vi "Termo_1.5__.vi"() -> ()   [LabVIEW 2015]
doc: "Программа мониторинга температуры"
panel:
  out "?":bool
  out "graph_update":bool
  out "Конфиг. АЦП?":bool
  in  "Tab Control":enum32{"ИЗМЕРЕНИЯ [К]", " АЦП", "ГРАФИК"}(tab)
  in  "T2_visible":bool=TRUE
  out "T6":dbl format="%.2f"
  in  "T5_visible":bool=TRUE
  out "R5":dbl format="%.2f"
  out "T3":dbl format="%.2f"
  out "R1":dbl format="%.2f"
  out "T2":dbl format="%.2f"
  out "T5":dbl format="%.2f"
  out "R3":dbl format="%.2f"
  out "T1":dbl format="%.2f"
  out "T4":dbl format="%.2f"
  out "R2":dbl format="%.2f"
  out "R4":dbl format="%.2f"
  out "R6":dbl format="%.2f"
  in  "T1_visible":bool=TRUE
  in  "T3_visible":bool=TRUE
  in  "T4_visible":bool=TRUE
  in  "T6_visible":bool=TRUE
  in  "stop":bool
  in  "ADC_dyn_range":T1(ring)=enum."± 0.625 В"
  in  "Buf_size":u8=1 min=1 max=128
  in  "SPS":T2(ring)
  in  "IP-адрес":string="10.10.10.65"
  in  "порт":u16=4001
  in  "Очистить график":bool
  in  "load_coeff.":bool caption="Disconn"
  in  "save_coeff.":bool caption="Disconn"
  in  "Coeff_cl_ch5":T3={"k1"=19.4736079181311652, "k2"=-232.79779903171584, "k3"=1229.13228608109057005, "k4"=-3103.0388431325554801, "k5"=4219.3520172238349901, "k6"=-2697.7160155214369299, "k7"=779.55193291697651198} caption="Канал 5" {"k7" format="%#_16g"; "k6" format="%#_16g"; "k5" format="%#_16g"; "k4" format="%#_16g"; "k3" format="%#_16g"; "k2" format="%#_16g"; "k1" format="%#_16g"}
  in  "Coeff_cl_ch6":T3={"k1"=11.9061392787261866, "k2"=-139.902402561856434, "k3"=774.882810204289854, "k4"=-1837.4832512177527, "k5"=2139.5822282396256899, "k6"=-730.555961686186492, "k7"=169.810834781266749} caption="Канал 6" {"k7" format="%#_16g"; "k6" format="%#_16g"; "k5" format="%#_16g"; "k4" format="%#_16g"; "k3" format="%#_16g"; "k2" format="%#_16g"; "k1" format="%#_16g"}
  in  "GraphLookB":bool
  in  "xScale -":bool
  in  "xScale +":bool
  out "мин.":string="1"
  in  "Старт измер.":bool
  in  "Стоп измер.":bool
  in  "Добавить время":dbl(ring)=300.0 items=["10 сек."=10.0, "1 мин."=60.0, "5 мин."=300.0, "20 мин."=1200.0]
  in  "Т min":dbl=4.0 min=-10.0 max=350.0 step=0.1
  in  "Т max":dbl=300.0 min=2.0 max=500.0 step=0.1
  out "часы":string="0"
  in  "Autoscale":bool=TRUE
  out "сек.":string="0"
  out "Сутки":string
  out "счетчик":u32=4001
  in  "Запись в файл":bool
  out "Path":string
  out "refnum out":refnum<file>
  in  "header?":bool caption="Disconn"
  out "con ID":refnum<k5>
  out "Graphs T":dynamicdata(graph) caption="ТЕМПЕРАТУРА, К"
  out "Расположение файла":path
  # "Т1"
  # "T2"
  # "Т3"
  # "Т4"
  # "Сопротивление, Ом"
  # "R1"
  # "R2"
  # "R3"
  # "R4"
  # "Скорость измерений"
  # "SPS = Samples Per Second"
  # "Размер буфера усреднения"
  # "Подключение"
  # "Шкала Т"
  # "Время графика"
  # ":"
  # ":"
  # "Измерения"
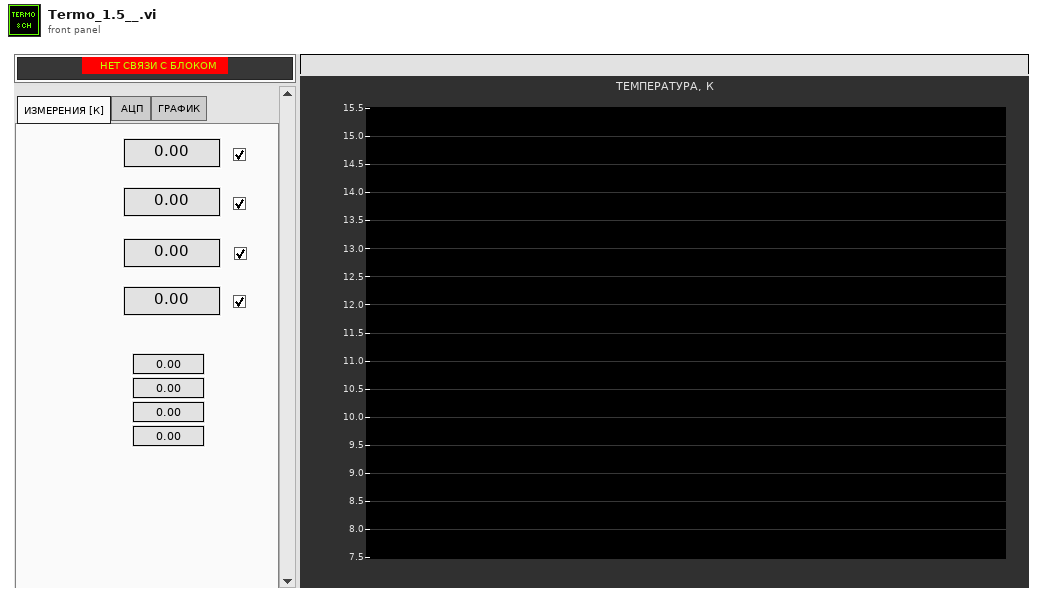
[diagram p1: front panel]
types:
  T1 = enum16{"± 5 В", "± 2.5 В", "± 1.25 В", "± 0.625 В", "± 312.5 мВ", "± 156.25 мВ", "± 78.125 мВ"}
  T2 = enum16{"2,5 SPS", "5 SPS", "10 SPS", "25 SPS", "50 SPS", "100 SPS", "500 SPS"}
  T3 = cluster{"k1":ext, "k2":ext, "k3":ext, "k4":ext, "k5":ext, "k6":ext, "k7":ext}
  T4 = enum32{"Page Enabled", "Page Disabled", "Page Disabled & Grayed"}
  T5 = enum16{"Standard", "Buffered", "CRLF", "Immediate"}
  T6 = cluster{"T1":dbl, " T2":dbl, " T3":dbl, "T4":dbl, "T5":dbl, "T6":dbl}
  T7 = typedef "LVDateTimeRec.ctl" = cluster{"fractional second":dbl, "second":i32, "minute":i32, "hour":i32, "day of month":i32, "month":i32, "year":i32, "day of week":i32, "day of year":i32, "DST":i32}
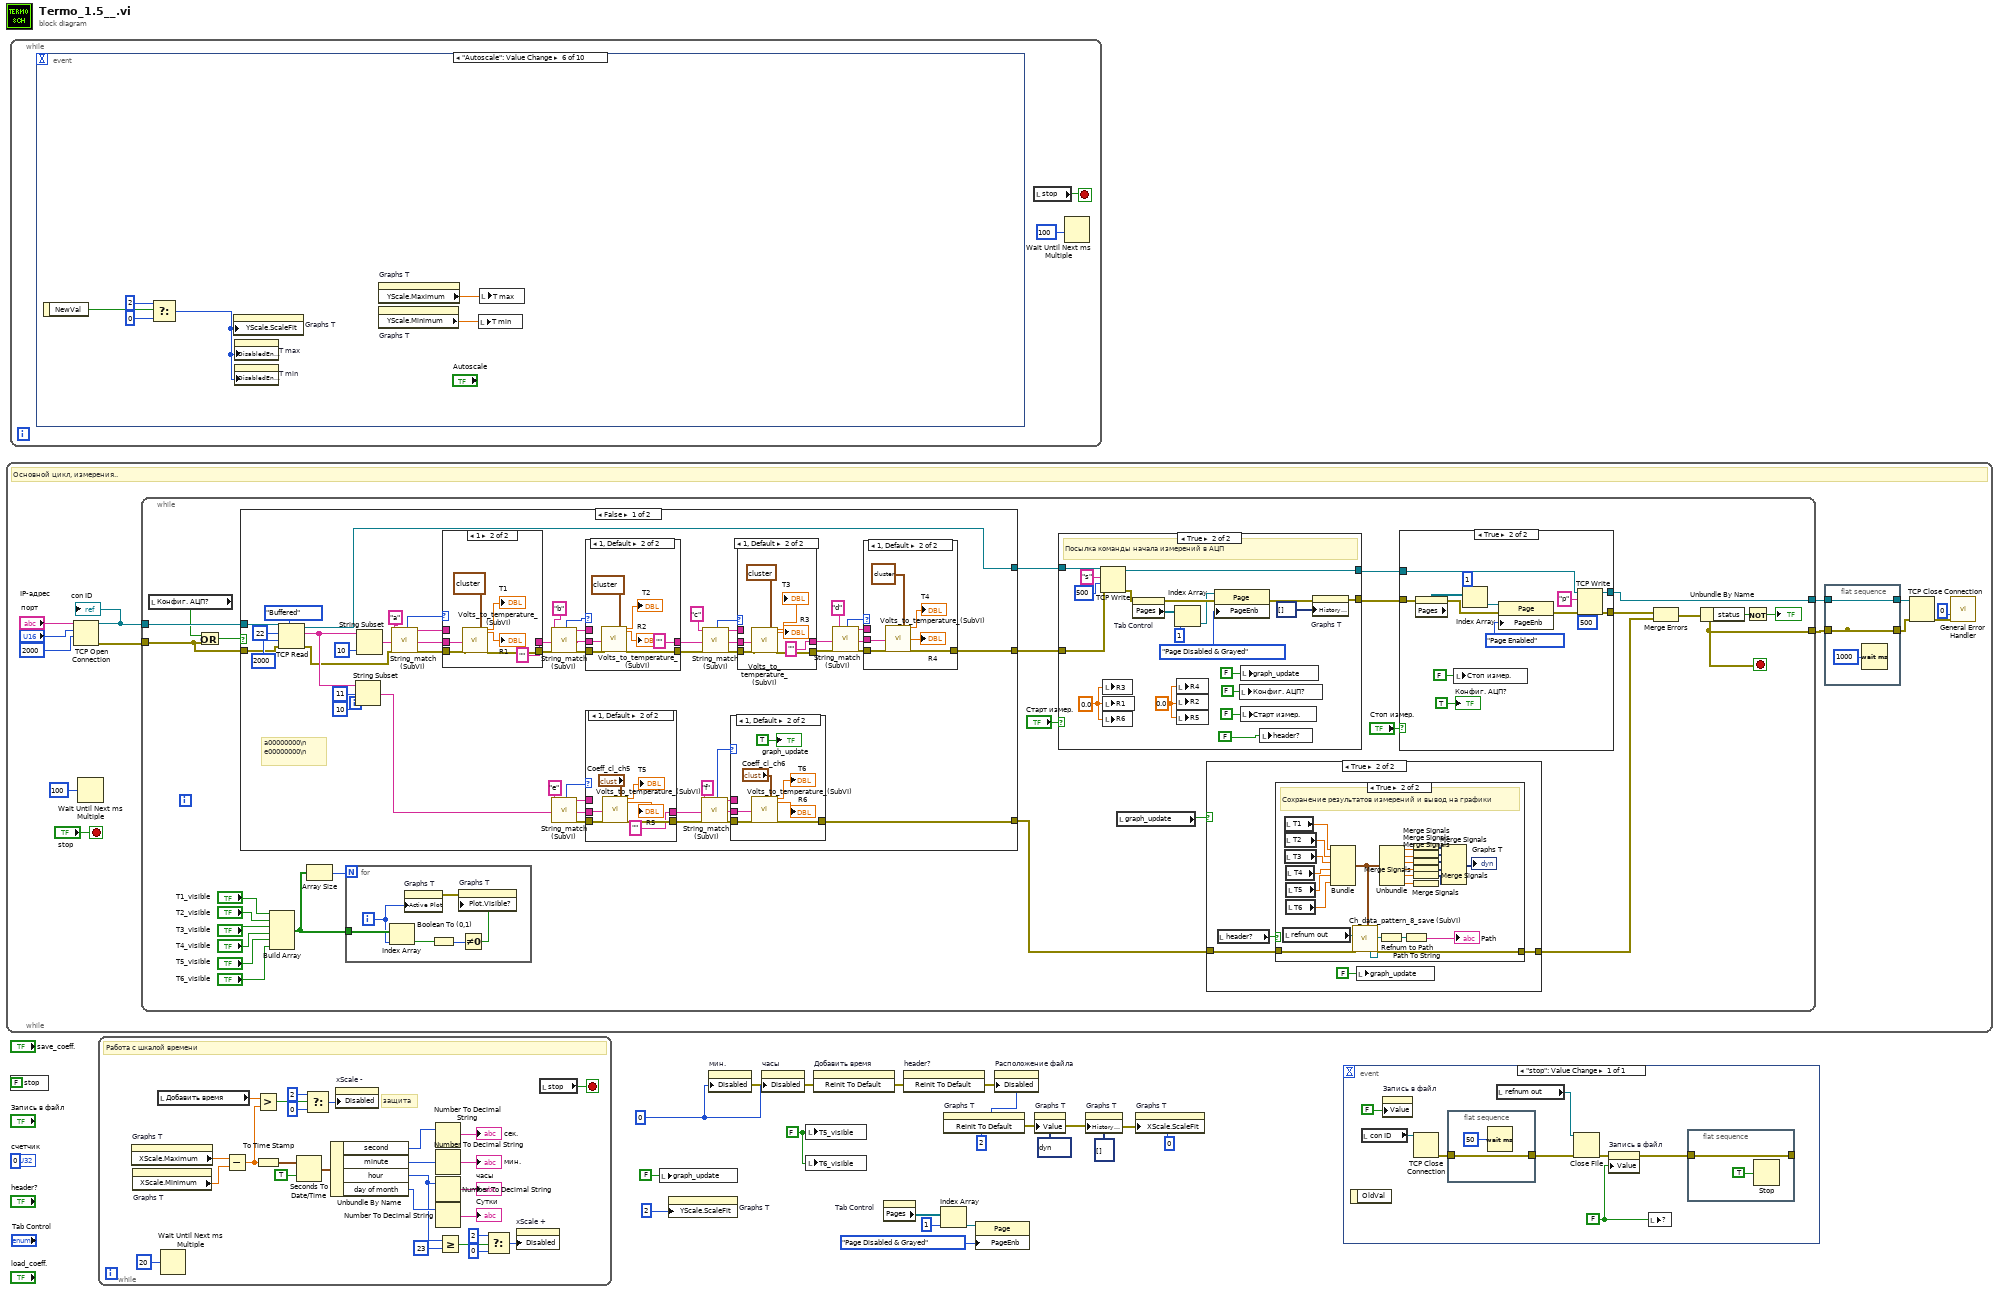
[diagram p0: block diagram]
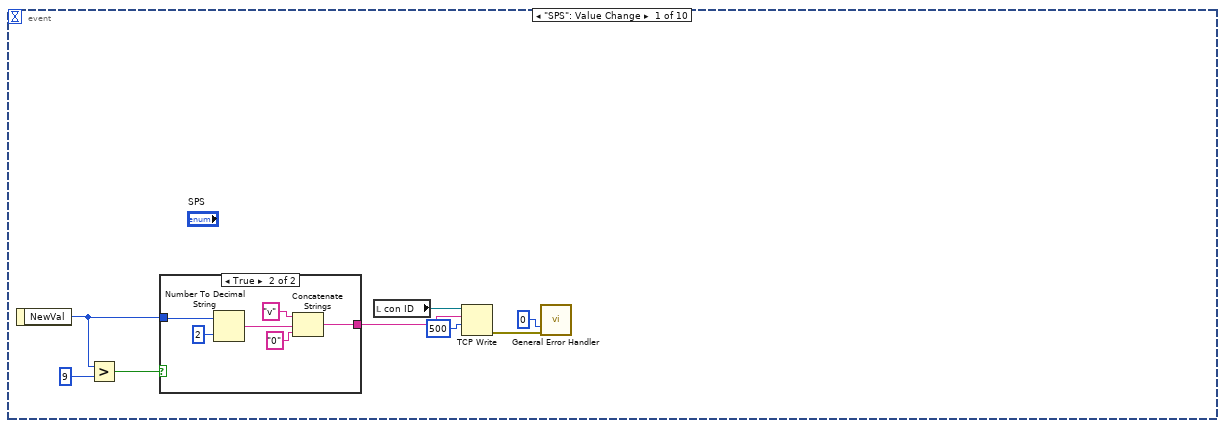
[diagram p2: hidden frame]
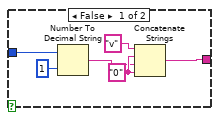
[diagram p3: hidden frame]
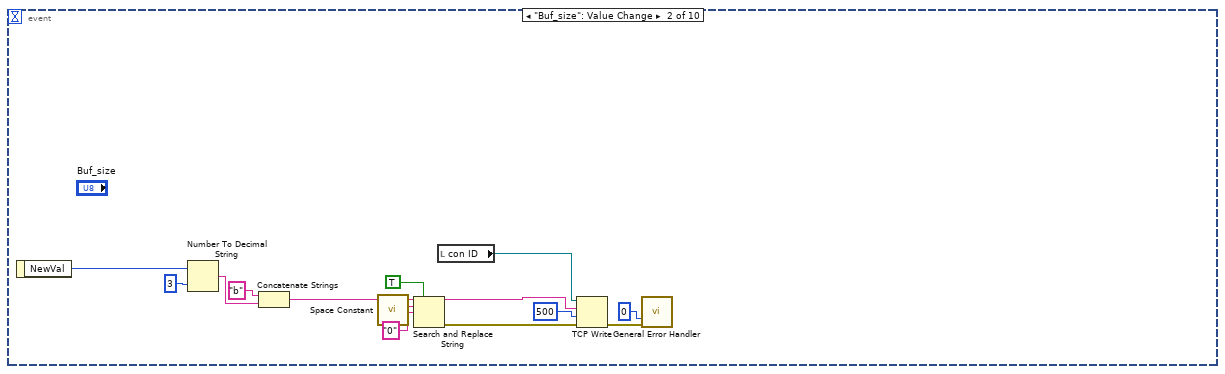
[diagram p4: hidden frame]
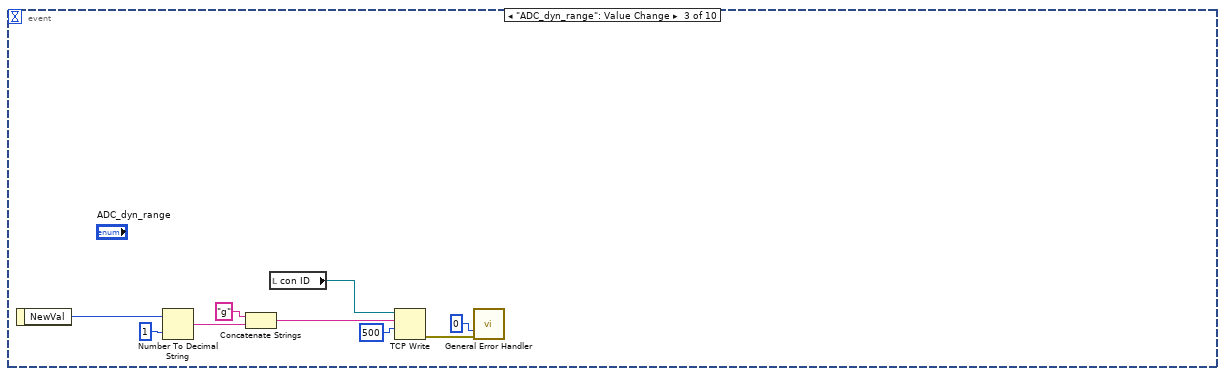
[diagram p5: hidden frame]
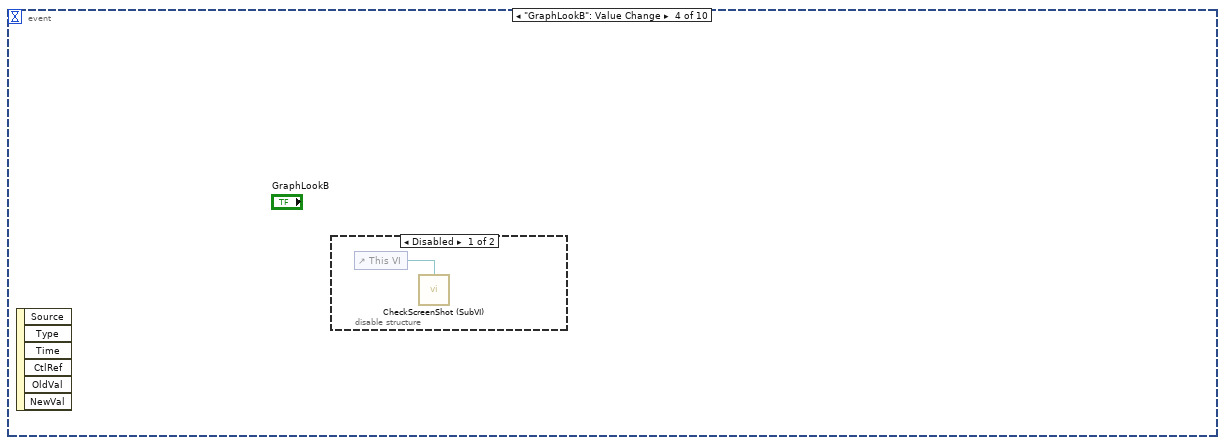
[diagram p6: hidden frame]
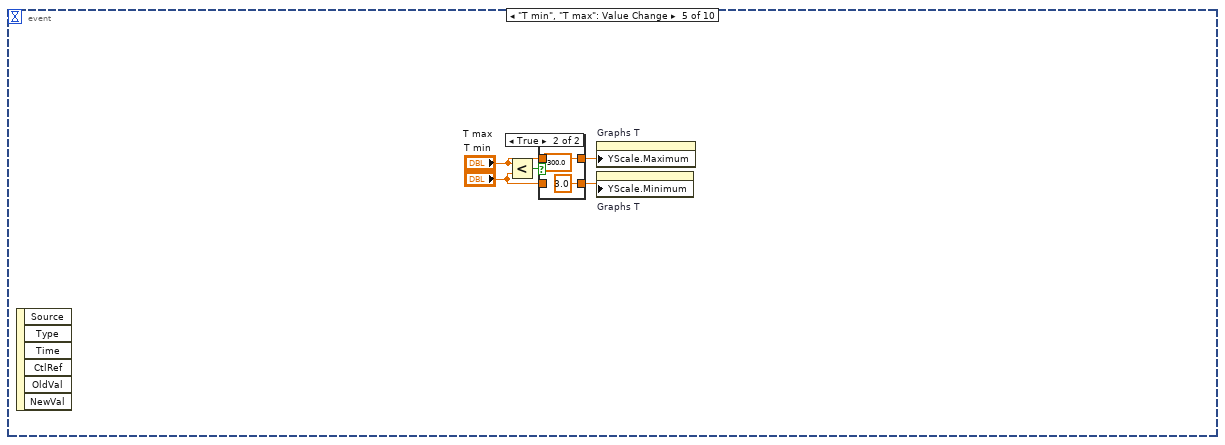
[diagram p8: hidden frame]
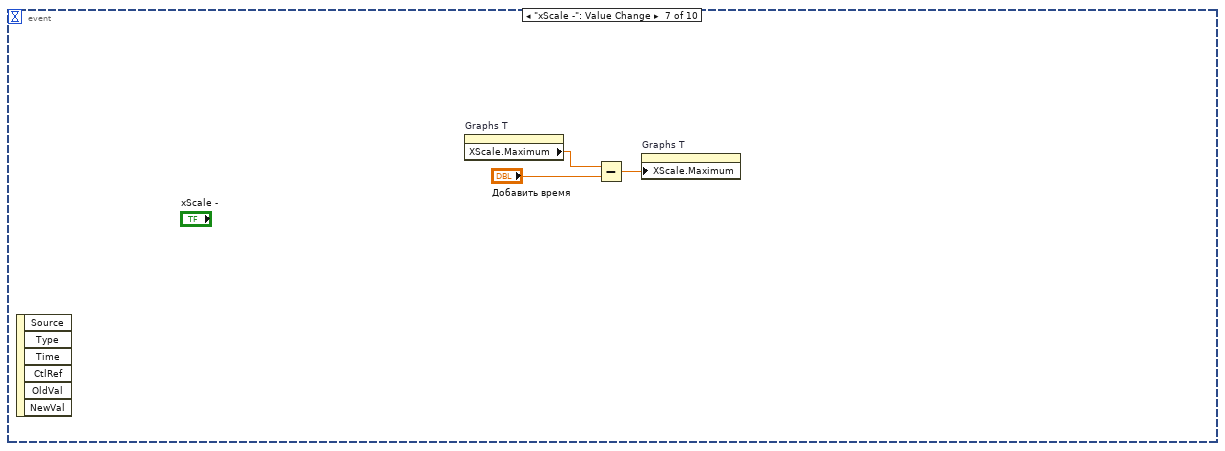
[diagram p10: hidden frame]
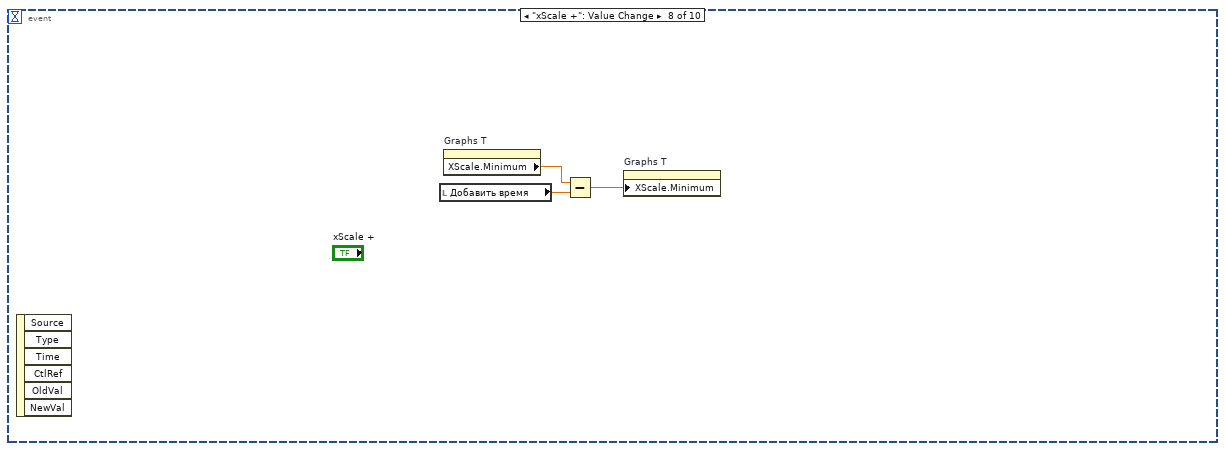
[diagram p11: hidden frame]
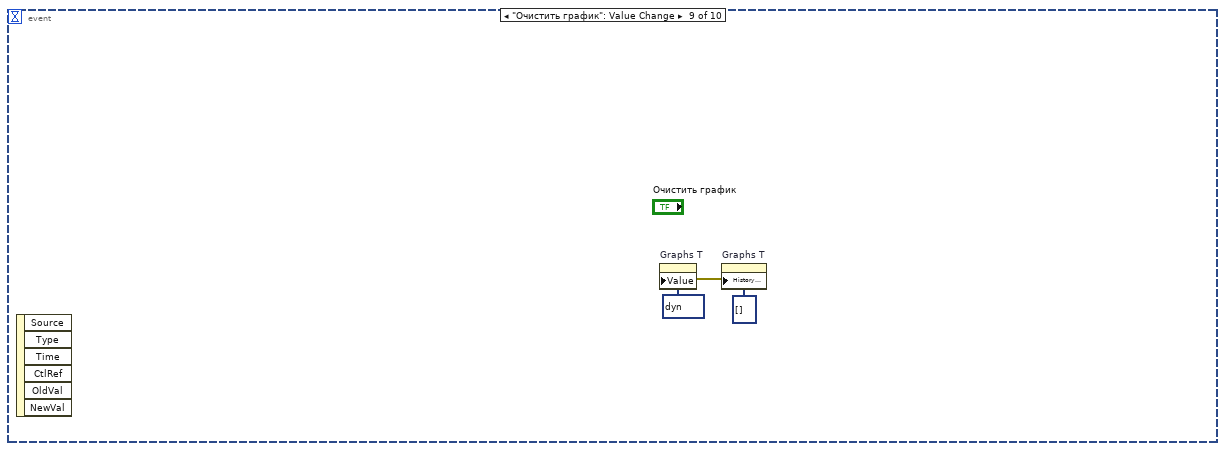
[diagram p12: hidden frame]
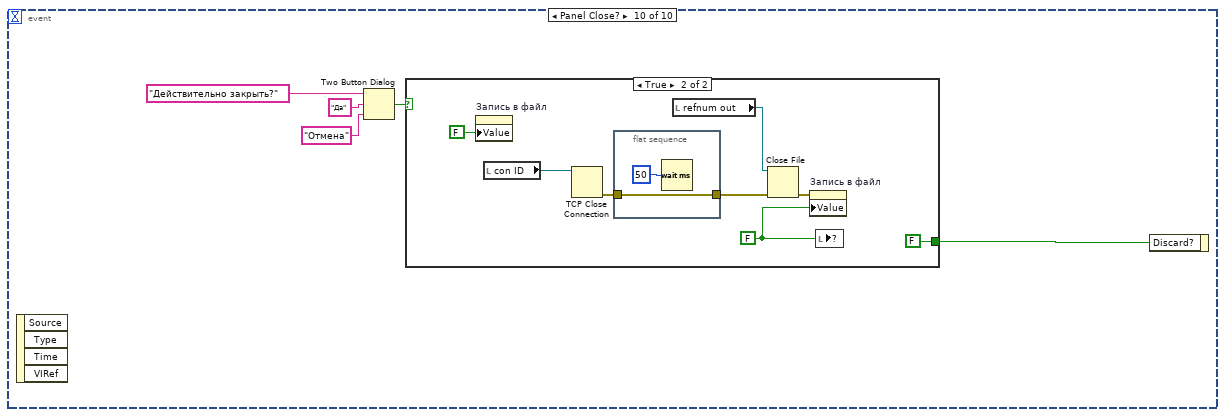
[diagram p13: hidden frame]
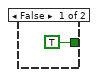
[diagram p14: hidden frame]
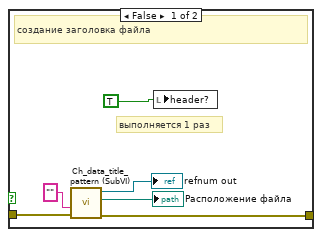
[diagram p16: hidden frame]
diagram:
  w1 = FALSE ("T5_visible")
  w20 = u8 0 ("Disabled")
  n1 = while {
    stop <- "stop" stop-if-true
    # "Основной цикл, измерения.."
    n2 = TCP Open Connection(address="IP-адрес", remote port or service name="порт", timeout ms (60000)=2000) -> (connection ID=w33:refnum<k5>, error out=w27:errorcluster)  [unwired: 1 in, 1 out]
    "con ID" <- w33
    n3 = Wait Until Next ms Multiple(millisecond multiple=u32 100) -> ()  [unwired: 1 out]
    n4 = while {
      tunnel: w33 -> [w63]
      tunnel: w27 -> [w46]
      tunnel: [w39] -> w25
      tunnel: [w38] -> w23
      stop <- w38 stop-if-true
      n5 = local read "Конфиг. АЦП?"() -> (w47:bool)
      n6 = Or(x=w47, y=w46) -> (x .or. y?=w61:bool)
      n7 = case shown="False" w61 {
        tunnel: [w146 w249] -> w48
        tunnel: w63 -> [w149 w249]
        tunnel: [w145 w248] -> w44
        tunnel: w46 -> [w147 w248]
        tunnel: [w144 _] -> w42
        frame False {
          # "a00000000\\n\ne00000000\\n"
          n8 = TCP Read(connection ID=w149, bytes to read=22, error in (no error)=w147, 7:T5."Buffered" ("mode (standard)"), 9:2000 ("timeout ms (25000)")) -> (connection ID out=w146:refnum<k5>, data out=w153:string, error out=w148:errorcluster)
          n9 = String Subset(string=w153, offset (0)=11, length (rest)=10 ("length (rest)")) -> (substring=w150:string)
          n10 = String Subset(string=w153, length (rest)=10 ("length (rest)")) -> (substring=w155:string)  [unwired: 1 in]
          n11 = call "String_match (SubVI).vi"("channel id"="a" ("regular expression"), "input string"=w155, "error in"=w148) -> ("match ?"=w161:i32, "output string"=w189:string, "match substring"=w190:string, "error out"=w191:errorcluster)  [unwired: 13 in]
          n12 = case shown="1" w161 {
            tunnel: [w240 w246] -> w180
            tunnel: w191 -> [w240 w247]
            tunnel: w190 -> [_ w245]
            tunnel: [w239 "" ("output string")] -> w193
            tunnel: w189 -> [w239 _]
            frame -1, Default {
            }
            frame 1 {
              n13 = call "Volts_to_temperature_(SubVI).vi"("ch_data_string"=w245, "error in"=w247, "koeff. cluster"=T3 {"k1"=130.445700915059999994, "k2"=-1315.82420889100000005, "k3"=5406.7587104216, "k4"=-11308.5781316600000004, "k5"=12719.274968733, "k6"=-7206.838528573, "k7"=1762.5796357467}) -> ("T solvation"=→"T1":dbl, "meas_voltage"=→"R1":dbl, "error out"=w246:errorcluster)  [unwired: 20 in, 2 out]
            }
          }
          n14 = call "String_match (SubVI).vi"("channel id"="b" ("regular expression"), "input string"=w193, "error in"=w180) -> ("match ?"=w160:i32, "output string"=w185:string, "match substring"=w186:string, "error out"=w187:errorcluster)  [unwired: 13 in]
          n15 = call "String_match (SubVI).vi"("channel id"="e" ("regular expression"), "input string"=w150) -> ("match ?"=w157:i32, "output string"=w178:string, "match substring"=w177:string, "error out"=w176:errorcluster)  [unwired: 14 in]
          n16 = case shown="1, Default" w160 {
            tunnel: [w231 w238] -> w169
            tunnel: w187 -> [w231 w237]
            tunnel: w186 -> [_ w236]
            tunnel: w185 -> [w230 _]
            tunnel: [w230 "" ("output string")] -> w168
            frame -1 {
            }
            frame 1, Default {
              n17 = call "Volts_to_temperature_(SubVI).vi"("ch_data_string"=w236, "error in"=w237, "koeff. cluster"=T3 {"k1"=158.97086338326, "k2"=-1680.987051628, "k3"=7248.2214480414, "k4"=-16012.25160649, "k5"=19138.901366204, "k6"=-11620.7677143299999996, "k7"=3012.5980224423}) -> ("T solvation"=→"T2":dbl, "meas_voltage"=→"R2":dbl, "error out"=w238:errorcluster)  [unwired: 20 in, 2 out]
            }
          }
          n18 = case shown="1, Default" w157 {
            tunnel: [w215 w222] -> w179
            tunnel: w176 -> [w215 w221]
            tunnel: w177 -> [_ w220]
            tunnel: [w214 "" ("output string")] -> w174
            tunnel: w178 -> [w214 _]
            frame -1 {
            }
            frame 1, Default {
              n19 = call "Volts_to_temperature_(SubVI).vi"("ch_data_string"=w220, "error in"=w221, "koeff. cluster"="Coeff_cl_ch5") -> ("T solvation"=→"T5":dbl, "meas_voltage"=→"R5":dbl, "error out"=w222:errorcluster)  [unwired: 20 in, 2 out]
            }
          }
          n20 = call "String_match (SubVI).vi"("channel id"="f" ("regular expression"), "input string"=w174, "error in"=w179) -> ("match ?"=w156:i32, "output string"=w173:string, "match substring"=w172:string, "error out"=w171:errorcluster)  [unwired: 13 in]
          n21 = call "String_match (SubVI).vi"("channel id"="c" ("regular expression"), "input string"=w168, "error in"=w169) -> ("match ?"=w159:i32, "output string"=w164:string, "match substring"=w165:string, "error out"=w166:errorcluster)  [unwired: 13 in]
          n22 = case shown="1, Default" w156 {
            tunnel: [w206 w213] -> w144
            tunnel: w171 -> [w206 w212]
            tunnel: w172 -> [_ w211]
            tunnel: w173 -> [_ _]
            frame -1 {
            }
            frame 1, Default {
              n23 = call "Volts_to_temperature_(SubVI).vi"("ch_data_string"=w211, "error in"=w212, "koeff. cluster"="Coeff_cl_ch6") -> ("T solvation"=→"T6":dbl, "meas_voltage"=→"R6":dbl, "error out"=w213:errorcluster)  [unwired: 20 in, 2 out]
              "graph_update" <- TRUE ("graph_update")
            }
          }
          n24 = case shown="1, Default" w159 {
            tunnel: w166 -> [w198 w205]
            tunnel: [w198 w204] -> w163
            tunnel: w165 -> [_ w202]
            tunnel: w164 -> [w197 _]
            tunnel: [w197 "" ("output string")] -> w162
            frame -1 {
            }
            frame 1, Default {
              n25 = call "Volts_to_temperature_(SubVI).vi"("ch_data_string"=w202, "error in"=w205, "koeff. cluster"=T3 {"k1"=18.933416559593, "k2"=-231.6963763814, "k3"=1256.05189673780000004, "k4"=-3242.759354941, "k5"=4499.4989483505, "k6"=-2910.138930261, "k7"=853.73352399654}) -> ("T solvation"=→"T3":dbl, "meas_voltage"=→"R3":dbl, "error out"=w204:errorcluster)  [unwired: 20 in, 2 out]
            }
          }
          n26 = call "String_match (SubVI).vi"("channel id"="d" ("regular expression"), "input string"=w162, "error in"=w163) -> ("match ?"=w158:i32, "output string"=w181:string, "match substring"=w182:string, "error out"=w183:errorcluster)  [unwired: 13 in]
          n27 = case shown="1, Default" w158 {
            tunnel: w183 -> [w223 w229]
            tunnel: [w223 w228] -> w145
            tunnel: w182 -> [_ w226]
            tunnel: w181 -> [_ _]
            frame -1 {
            }
            frame 1, Default {
              n28 = call "Volts_to_temperature_(SubVI).vi"("ch_data_string"=w226, "error in"=w229, "koeff. cluster"=T3 {"k1"=-1.22849768937512731, "k2"=42.2580823609605432, "k3"=-271.179135338868946, "k4"=1161.17997252382338, "k5"=-2451.5718683190643801, "k6"=2722.134789723902, "k7"=-982.529668014}) -> ("T solvation"=→"T4":dbl, "meas_voltage"=→"R4":dbl, "error out"=w228:errorcluster)  [unwired: 20 in, 2 out]
            }
          }
        }
        frame True {
        }
      }
      n29 = Build Array("T1_visible", "T2_visible", "T3_visible", "T4_visible", "T5_visible", "T6_visible") -> (w53:bool[])
      n30 = Array Size(array=w53) -> (size(s)=w54:i32)
      n31 = for {
        N: w54 -> [_]
        tunnel: w53 -> [w142]
        i -> [w140]
        n32 = Index Array(array=w142, index=w140) -> (element=w139:bool)
        n33 = property on="Graphs T" class="WFChart (strict)"("Active Plot"=w140) -> (error out=w141:errorcluster)  [unwired: 2 in, 1 out]
        n34 = Boolean To (0,1)(Boolean=w139) -> (0, 1=w143:i16)
        n35 = Not Equal To 0?(x=w143) -> (x != 0?=w138:bool)
        n36 = property on="Graphs T" class="WFChart (strict)"(error in=w141, "Plot.Visible?"=w138) -> ()  [unwired: 1 in, 2 out]
      }
      n37 = case shown="True" "Старт измер." {
        tunnel: [w116 w127] -> w50
        tunnel: [w117 w126] -> w52
        tunnel: w48 -> [w117 w121]
        tunnel: w44 -> [w116 w120]
        frame False {
        }
        frame True {
          w123 = 0.0 ("3")
          w118 = 0.0 ("3")
          # "Посылка команды начала измерений в АЦП"
          n38 = TCP Write(connection ID=w121, data in="s", error in (no error)=w120, 9:500 ("timeout ms (25000)")) -> (connection ID out=w126:refnum<k5>, error out=w135:errorcluster)  [unwired: 1 out]
          n39 = local write "R3"(w118) -> ()
          n40 = local write "R1"(w118) -> ()
          n41 = local write "R6"(w118) -> ()
          n42 = property on="Tab Control" class="TabCtl (strict)"(error in=w135) -> (error out=w136:errorcluster, "Pages"=w131:refnum<vi>[])  [unwired: 1 in, 1 out]
          n43 = Index Array(array=w131, index=1) -> (element=w132:refnum<vi>)
          n44 = local write "R4"(w123) -> ()
          n45 = local write "R2"(w123) -> ()
          n46 = local write "R5"(w123) -> ()
          n47 = property class="Page"(reference=w132, error in=w136, "PageEnb"=T4."Page Disabled & Grayed" ("Page Enabled State")) -> (error out=w122:errorcluster)  [unwired: 1 out]
          n48 = local write "Конфиг. АЦП?"(FALSE ("Старт измер.")) -> ()
          n49 = local write "graph_update"(FALSE ("graph_update")) -> ()
          n50 = local write "Старт измер."(FALSE ("Старт измер.")) -> ()
          n51 = local write "header?"(FALSE ("flag1")) -> ()
          n52 = property on="Graphs T" class="WFChart (strict)"(error in=w122, "History Data"=dynamicdata[] []) -> (error out=w127:errorcluster)  [unwired: 1 in, 1 out]
        }
      }
      n53 = local read "graph_update"() -> (w43:bool)
      n54 = case shown="True" w43 {
        tunnel: w42 -> [w64 w66]
        tunnel: [w64 w65] -> w40
        frame False {
        }
        frame True {
          n55 = local read "header?"() -> (w68:bool)
          n56 = case shown="True" w68 {
            tunnel: w66 -> [w69 w83]
            tunnel: [w71 w82] -> w65
            frame False {
              # "выполняется 1 раз"
              # "создание заголовка файла"
              n57 = call "Ch_data_title_pattern (SubVI).vi"("error in"=w69, "Единица измерений"="") -> ("error out"=w71:errorcluster, "Path"=→"Расположение файла":path, "Byte Stream File out"=→"refnum out":refnum<file>)  [unwired: 7 in]
              n58 = local write "header?"(TRUE ("flag1")) -> ()
            }
            frame True {
              # "Сохранение результатов измерений и вывод на графики"
              n59 = local read "refnum out"() -> (w81:refnum<file>)
              n60 = local read "T1"() -> (w80:dbl)
              n61 = local read "T2"() -> (w79:dbl)
              n62 = local read "T3"() -> (w78:dbl)
              n63 = local read "T4"() -> (w77:dbl)
              n64 = local read "T5"() -> (w76:dbl)
              n65 = local read "T6"() -> (w75:dbl)
              n66 = Bundle("T1"=w80, "T2"=w79, "T3"=w78, "T4"=w77, "T5"=w76, "T6"=w75) -> (w99:T6)  [unwired: 1 in]
              n67 = call "Ch_data_pattern_8_save (SubVI).vi"("error in"=w83, "T Cluster"=w99, "file"=w81) -> ("error out"=w82:errorcluster)  [unwired: 24 in]
              n68 = Refnum to Path(1:w81) -> (0:w98:path)
              n69 = Unbundle(w99) -> ("T1"=w91:dbl, "T2"=w90:dbl, "T3"=w89:dbl, "T4"=w88:dbl, "T5"=w86:dbl, "T6"=w84:dbl)
              n70 = Path To String(path=w98) -> (string=→"Path":string)
              n71 = Merge Signals(w91) -> (w94:dynamicdata)
              n72 = Merge Signals(w90) -> (w95:dynamicdata)
              n73 = Merge Signals(w89) -> (w96:dynamicdata)
              n74 = Merge Signals(w88) -> (w93:dynamicdata)
              n75 = Merge Signals(w86) -> (w87:dynamicdata)
              n76 = Merge Signals(w84) -> (w85:dynamicdata)
              n77 = Merge Signals(w94, w95, w96, w93, w87, w85) -> (→"Graphs T":dynamicdata)
            }
          }
          n78 = local write "graph_update"(FALSE ("graph_update")) -> ()
        }
      }
      n79 = case shown="True" "Стоп измер." {
        tunnel: w50 -> [w100 w108]
        tunnel: w52 -> [w101 w106]
        tunnel: [w100 w102] -> w41
        tunnel: [w101 w103] -> w39
        frame False {
        }
        frame True {
          n80 = property on="Tab Control" class="TabCtl (strict)"(error in=w108) -> (error out=w107:errorcluster, "Pages"=w111:refnum<vi>[])  [unwired: 1 in, 1 out]
          n81 = local write "Стоп измер."(FALSE ("Стоп измер.")) -> ()
          n82 = Index Array(array=w111, index=1) -> (element=w112:refnum<vi>)
          n83 = property class="Page"(reference=w112, error in=w107, "PageEnb"=T4."Page Enabled" ("Page Enabled State")) -> (error out=w115:errorcluster)  [unwired: 1 out]
          n84 = TCP Write(connection ID=w106, data in="p", error in (no error)=w115, 9:500 ("timeout ms (25000)")) -> (connection ID out=w103:refnum<k5>, error out=w102:errorcluster)  [unwired: 1 out]
          "Конфиг. АЦП?" <- TRUE ("Конфиг. АЦП?")
        }
      }
      n85 = Merge Errors(w41, w40) -> (w38:errorcluster)
      n86 = Unbundle By Name(w38) -> ("status"=w45:bool)
      n87 = Not(x=w45) -> (.not. x?=→"?":bool)
    }
    n88 = flat-sequence {
      tunnel: [w36] -> w24
      tunnel: w25 -> [w36]
      tunnel: w23 -> [w35]
      tunnel: [w35] -> _
      tunnel: [w35] -> w22
      frame #0 {
        n89 = Wait (ms)(milliseconds to wait=u32 1000) -> ()  [unwired: 1 out]
      }
    }
    n90 = TCP Close Connection(connection ID=w24, error in (no error)=w22) -> (error out=w32:errorcluster)  [unwired: 2 out]
    n91 = call <vilib>:"General Error Handler.vi"("type of dialog (OK msg:1)"=u32 0 ("milliseconds to wait"), "error in (no error)"=w32) -> ()  [unwired: 1 in, 13 out]
  }
  n92 = while {
    stop <- w250 stop-if-true
    n93 = event shown="[5] \"Autoscale\": Value Change" {
      selector: _ -> [_ _ _ _ _ _ _ _ _ _]
      dyn-events: _ -> [_ _ _ _ _ _ _ _ _ _]
      timeout: _ -> [_ _ _ _ _ _ _ _ _ _]
      event "SPS": Value Change {
        n94 = event-data() -> ("NewVal"=w255:T2)  [unwired: 1 in]
        n95 = Greater?(x=w255, y=9 ("timeout ms (25000)")) -> (0:w253:bool)
        n96 = case shown="True" w253 {
          tunnel: w255 -> [w265 w271]
          tunnel: [w262 w266] -> w252
          frame False {
            w261 = "0" ("string")
            n97 = Number To Decimal String(number=w265, width (-)=i16 1) -> (decimal integer string=w260:string)
            n98 = Concatenate Strings("v" ("data in"), w261, w260, w261) -> (w262:string)
          }
          frame True {
            n99 = Number To Decimal String(number=w271, width (-)=i16 2) -> (decimal integer string=w268:string)
            n100 = Concatenate Strings("v" ("data in"), w268, "0" ("string")) -> (w266:string)
          }
        }
        n101 = local read "con ID"() -> (w258:refnum<k5>)
        n102 = TCP Write(connection ID=w258, data in=w252, 9:500 ("timeout ms (25000)")) -> (error out=w257:errorcluster)  [unwired: 1 in, 2 out]
        n103 = call <vilib>:"General Error Handler.vi"("type of dialog (OK msg:1)"=0 ("timeout ms (25000)"), "error in (no error)"=w257) -> ()  [unwired: 9 in, 5 out]
      }
      event "Buf_size": Value Change {
        n104 = event-data() -> ("NewVal"=w282:u8)  [unwired: 1 in]
        n105 = Number To Decimal String(number=w282, width (-)=i16 3) -> (decimal integer string=w280:string)
        n106 = Concatenate Strings("b" ("data in"), w280) -> (w279:string)
        n107 = call <vilib>:"Space Constant.vi"() -> ("String"=w277:string)
        n108 = Search and Replace String(replace all?=TRUE ("replace all? (F)"), input string=w279, search string=w277, replace string="0" ("replace string (\"\")")) -> (result string=w278:string, error out=w274:errorcluster)  [unwired: 4 in, 2 out]
        n109 = local read "con ID"() -> (w284:refnum<k5>)
        n110 = TCP Write(connection ID=w284, data in=w278, error in (no error)=w274, 9:500 ("timeout ms (25000)")) -> (error out=w273:errorcluster)  [unwired: 2 out]
        n111 = call <vilib>:"General Error Handler.vi"("type of dialog (OK msg:1)"=0 ("timeout ms (25000)"), "error in (no error)"=w273) -> ()  [unwired: 9 in, 5 out]
      }
      event "ADC_dyn_range": Value Change {
        n112 = event-data() -> ("NewVal"=w291:T1)  [unwired: 1 in]
        n113 = Number To Decimal String(number=w291, width (-)=i16 1) -> (decimal integer string=w289:string)
        n114 = Concatenate Strings("g" ("data in"), w289) -> (w288:string)
        n115 = local read "con ID"() -> (w293:refnum<k5>)
        n116 = TCP Write(connection ID=w293, data in=w288, 9:500 ("timeout ms (25000)")) -> (error out=w286:errorcluster)  [unwired: 1 in, 2 out]
        n117 = call <vilib>:"General Error Handler.vi"("type of dialog (OK msg:1)"=0 ("timeout ms (25000)"), "error in (no error)"=w286) -> ()  [unwired: 9 in, 5 out]
      }
      event "GraphLookB": Value Change {
        n118 = event-data() -> ()  [unwired: 1 in, 6 out]
        n119 = disable-structure shown="Disabled" {
          frame Disabled {
            n120 = control-ref of="This VI"() -> (w295:refnum<vi>)
            n121 = call "CheckScreenShot (SubVI).vi"("VI reference"=w295) -> ()  [unwired: 15 in]
          }
          frame Enabled {
          }
        }
      }
      event "Т min", "Т max": Value Change {
        n122 = event-data() -> ()  [unwired: 1 in, 6 out]
        n123 = Less?(x="Т max", y="Т min") -> (x < y?=w296:bool)
        n124 = case shown="True" w296 {
          tunnel: [w301 300.0 ("x+1")] -> w298
          tunnel: [w302 3.0 ("x+1")] -> w297
          tunnel: "Т max" -> [w301 _]
          tunnel: "Т min" -> [w302 _]
          frame False {
          }
          frame True {
          }
        }
        n125 = property on="Graphs T" class="WFChart (strict)"("YScale.Maximum"=w298) -> ()  [unwired: 2 in, 2 out]
        n126 = property on="Graphs T" class="WFChart (strict)"("YScale.Minimum"=w297) -> ()  [unwired: 2 in, 2 out]
      }
      event "Autoscale": Value Change {
        n127 = event-data() -> ("NewVal"=w305:bool)  [unwired: 1 in]
        n128 = Select(t=u8 2 ("Y Scale.Scale Fit"), s=w305, f=u8 0 ("Y Scale.Scale Fit")) -> (s? t:f=w308:u8)
        n129 = property on="Graphs T" class="WFChart (strict)"("YScale.ScaleFit"=w308) -> ()  [unwired: 2 in, 2 out]
        n130 = property on="Т max" class="DigNum (strict)"("DisabledEnum"=w308) -> ()  [unwired: 2 in, 2 out]
        n131 = property on="Т min" class="DigNum (strict)"("DisabledEnum"=w308) -> ()  [unwired: 2 in, 2 out]
        n132 = property on="Graphs T" class="WFChart (strict)"() -> ("YScale.Maximum"=w306:dbl)  [unwired: 2 in, 2 out]
        n133 = property on="Graphs T" class="WFChart (strict)"() -> ("YScale.Minimum"=w307:dbl)  [unwired: 2 in, 2 out]
        n134 = local write "Т min"(w307) -> ()
        n135 = local write "Т max"(w306) -> ()
      }
      event "xScale -": Value Change {
        n136 = event-data() -> ()  [unwired: 1 in, 6 out]
        n137 = property on="Graphs T" class="WFChart (strict)"() -> ("XScale.Maximum"=w313:dbl)  [unwired: 2 in, 2 out]
        n138 = Subtract(x=w313, y="Добавить время") -> (x-y=w312:dbl)
        n139 = property on="Graphs T" class="WFChart (strict)"("XScale.Maximum"=w312) -> ()  [unwired: 2 in, 2 out]
      }
      event "xScale +": Value Change {
        n140 = event-data() -> ()  [unwired: 1 in, 6 out]
        n141 = local read "Добавить время"() -> (w314:dbl)
        n142 = property on="Graphs T" class="WFChart (strict)"() -> ("XScale.Minimum"=w316:dbl)  [unwired: 2 in, 2 out]
        n143 = Subtract(x=w316, y=w314) -> (x-y=w315:dbl)
        n144 = property on="Graphs T" class="WFChart (strict)"("XScale.Minimum"=w315) -> ()  [unwired: 2 in, 2 out]
      }
      event "Очистить график": Value Change {
        n145 = event-data() -> ()  [unwired: 1 in, 6 out]
        n146 = property on="Graphs T" class="WFChart (strict)"("Value"=dynamicdata [{"t0"=timestamp(3465273261.7246556 s since 1904-01-01), "dt"=1.0, "Y"=[0.1931097262457384]}, {"t0"=timestamp(3465273261.7246556 s since 1904-01-01), "dt"=1.0, "Y"=[0.3594116459482981]}, {"t0"=timestamp(3465273261.7246556 s since 1904-01-01), "dt"=1.0, "Y"=[0.8898205452798131]}, {"t0"=timestamp(3465273261.7246556 s since 1904-01-01), "dt"=1.0, "Y"=[0.747699236883661]}] ("Graphs")) -> (error out=w318:errorcluster)  [unwired: 2 in, 1 out]
        n147 = property on="Graphs T" class="WFChart (strict)"(error in=w318, "History Data"=dynamicdata[] []) -> ()  [unwired: 1 in, 2 out]
      }
      event Panel Close? {
        n148 = event-data() -> ()  [unwired: 1 in, 4 out]
        n149 = Two Button Dialog(message="Действительно закрыть?", 1:"Отмена" ("T button name (\"OK\")"), 2:"Да" ("T button name (\"OK\")")) -> (T button?=w321:bool)
        n150 = case shown="True" w321 {
          tunnel: [TRUE ("Discard?") FALSE ("Discard?")] -> w320
          frame False {
          }
          frame True {
            w330 = FALSE ("Запись в файл")
            n151 = property on="Запись в файл" class="Bool (strict)"("Value"=FALSE ("Запись в файл")) -> ()  [unwired: 2 in, 2 out]
            n152 = local read "con ID"() -> (w327:refnum<k5>)
            n153 = TCP Close Connection(connection ID=w327) -> (error out=w333:errorcluster)  [unwired: 1 in, 2 out]
            n154 = flat-sequence {
              tunnel: [w334] -> w332
              tunnel: w333 -> [w334]
              frame #0 {
                n155 = Wait (ms)(milliseconds to wait=u32 50) -> ()  [unwired: 1 out]
              }
            }
            n156 = local read "refnum out"() -> (w329:refnum<file>)
            n157 = Close File(refnum=w329, error in=w332) -> (error out=w328:errorcluster)  [unwired: 1 out]
            n158 = property on="Запись в файл" class="Bool (strict)"(error in=w328, "Value"=w330) -> ()  [unwired: 1 in, 2 out]
            n159 = local write item#8(w330) -> ()
          }
        }
        n160 = event-data("Discard?"=w320) -> ()  [unwired: 1 in, 1 out]
      }
    }
    n161 = local read "stop"() -> (w250:bool)
    n162 = Wait Until Next ms Multiple(millisecond multiple=u32 100 ("milliseconds to wait")) -> ()  [unwired: 1 out]
  }
  n163 = local write "stop"(FALSE ("Boolean")) -> ()
  n164 = while {
    stop <- w361 stop-if-true
    # "защита"
    # "Работа с шкалой времени"
    n165 = property on="Graphs T" class="WFChart (strict)"() -> ("XScale.Maximum"=w337:dbl)  [unwired: 2 in, 2 out]
    n166 = property on="Graphs T" class="WFChart (strict)"() -> ("XScale.Minimum"=w336:dbl)  [unwired: 2 in, 2 out]
    n167 = local read "Добавить время"() -> (w360:dbl)
    n168 = Wait Until Next ms Multiple(millisecond multiple=u32 20) -> ()  [unwired: 1 out]
    n169 = Subtract(x=w337, y=w336) -> (x-y=w350:dbl)
    n170 = Greater?(x=w360, y=w350) -> (0:w343:bool)
    n171 = To Time Stamp(1:w350) -> (0:w358:timestamp)
    n172 = Seconds To Date/Time(time stamp (now)=w358, to UTC (F)=TRUE) -> (date time rec=w357:T7)
    n173 = Select(t=u8 2 ("Disabled"), s=w343, f=u8 0 ("Disabled")) -> (s? t:f=w346:u8)
    n174 = Unbundle By Name(w357) -> ("second"=w356:i32, "minute"=w355:i32, "hour"=w348:i32, "day of month"=w354:i32)
    n175 = property on="xScale -" class="Bool (strict)"("Disabled"=w346) -> ()  [unwired: 2 in, 2 out]
    n176 = Number To Decimal String(number=w356) -> (decimal integer string=→"сек.":string)  [unwired: 1 out]
    n177 = Number To Decimal String(number=w355) -> (decimal integer string=→"мин.":string)  [unwired: 1 out]
    n178 = Number To Decimal String(number=w348) -> (decimal integer string=→"часы":string)  [unwired: 1 out]
    n179 = Number To Decimal String(number=w354) -> (decimal integer string=→"Сутки":string)  [unwired: 1 out]
    n180 = Greater Or Equal?(x=w348, y=23) -> (x >= y?=w339:bool)
    n181 = Select(t=u8 2 ("Disabled"), s=w339, f=u8 0 ("Disabled")) -> (s? t:f=w342:u8)
    n182 = property on="xScale +" class="Bool (strict)"("Disabled"=w342) -> ()  [unwired: 2 in, 2 out]
    n183 = local read "stop"() -> (w361:bool)
  }
  n184 = local write "graph_update"(FALSE ("graph_update")) -> ()
  n185 = property on="Graphs T" class="WFChart (strict)"("YScale.ScaleFit"=u8 2 ("Y Scale.Scale Fit")) -> ()  [unwired: 2 in, 2 out]
  n186 = property on="мин." class="Str"("Disabled"=w20) -> (error out=w19:errorcluster)  [unwired: 2 in, 1 out]
  n187 = property on="часы" class="Str"(error in=w19, "Disabled"=w20) -> (error out=w18:errorcluster)  [unwired: 1 in, 1 out]
  n188 = local write "T5_visible"(w1) -> ()
  n189 = local write "T6_visible"(w1) -> ()
  n190 = invoke on="Добавить время" class="Ring (strict)" method="Reinit To Default"(error in=w18) -> (error out=w12:errorcluster)  [unwired: 2 in, 2 out]
  n191 = property on="Tab Control" class="TabCtl (strict)"() -> ("Pages"=w13:refnum<vi>[])  [unwired: 2 in, 2 out]
  n192 = invoke on="header?" class="Bool (strict)" method="Reinit To Default"(error in=w12) -> (error out=w17:errorcluster)  [unwired: 2 in, 2 out]
  n193 = Index Array(array=w13, index=1) -> (element=w14:refnum<vi>)
  n194 = invoke on="Graphs T" class="WFChart (strict)" method="Reinit To Default"() -> (error out=w9:errorcluster)  [unwired: 3 in, 2 out]
  n195 = property class="Page"(reference=w14, "PageEnb"=T4."Page Disabled & Grayed" ("Page Enabled State")) -> ()  [unwired: 1 in, 2 out]
  n196 = property on="Расположение файла" class="Path"(error in=w17, "Disabled"=u8 2) -> ()  [unwired: 1 in, 2 out]
  n197 = property on="Graphs T" class="WFChart (strict)"(error in=w9, "Value"=dynamicdata [{"t0"=timestamp(3465273261.7246556 s since 1904-01-01), "dt"=1.0, "Y"=[0.1931097262457384]}, {"t0"=timestamp(3465273261.7246556 s since 1904-01-01), "dt"=1.0, "Y"=[0.3594116459482981]}, {"t0"=timestamp(3465273261.7246556 s since 1904-01-01), "dt"=1.0, "Y"=[0.8898205452798131]}, {"t0"=timestamp(3465273261.7246556 s since 1904-01-01), "dt"=1.0, "Y"=[0.747699236883661]}] ("Graphs")) -> (error out=w8:errorcluster)  [unwired: 1 in, 1 out]
  n198 = property on="Graphs T" class="WFChart (strict)"(error in=w8, "History Data"=dynamicdata[] []) -> (error out=w11:errorcluster)  [unwired: 1 in, 1 out]
  n199 = property on="Graphs T" class="WFChart (strict)"(error in=w11, "XScale.ScaleFit"=u8 0 ("Y Scale.Scale Fit")) -> ()  [unwired: 1 in, 2 out]
  n200 = event shown="[0] \"stop\": Value Change" {
    selector: _ -> [_]
    dyn-events: _ -> [_]
    timeout: _ -> [_]
    event "stop": Value Change {
      w366 = FALSE ("Запись в файл")
      n201 = event-data() -> ()  [unwired: 1 in, 1 out]
      n202 = local read "con ID"() -> (w363:refnum<k5>)
      n203 = property on="Запись в файл" class="Bool (strict)"("Value"=FALSE ("Запись в файл")) -> ()  [unwired: 2 in, 2 out]
      n204 = TCP Close Connection(connection ID=w363) -> (error out=w369:errorcluster)  [unwired: 1 in, 2 out]
      n205 = flat-sequence {
        tunnel: [w372] -> w368
        tunnel: w369 -> [w372]
        frame #0 {
          n206 = Wait (ms)(milliseconds to wait=u32 50) -> ()  [unwired: 1 out]
        }
      }
      n207 = local read "refnum out"() -> (w365:refnum<file>)
      n208 = Close File(refnum=w365, error in=w368) -> (error out=w364:errorcluster)  [unwired: 1 out]
      n209 = property on="Запись в файл" class="Bool (strict)"(error in=w364, "Value"=w366) -> (error out=w362:errorcluster)  [unwired: 1 in, 1 out]
      n210 = local write item#8(w366) -> ()
      n211 = flat-sequence {
        tunnel: w362 -> [w371]
        tunnel: [w371] -> _
        frame #0 {
          n212 = Stop(stop? (T)=TRUE) -> ()
        }
      }
    }
  }
  "счетчик" <- u32 0 ("счетчик")
